vi "Global_Pictures.vi"() -> ()   [LabVIEW 2010]
panel:
  in  "sw PF Dir":bool[](array[boolean])
  in  "Tr PF Dir":bool[](array[boolean])
  in  "Line PF Dir":bool[](array[boolean])
  in  "Selection":bool
  in  "Zoom Delta":dbl
  in  "Layer History":string[](array[string])
  in  "Selected Layer":string
  out "ColorScale":picture
  in  "Tr Colors":u32[](array[colorbox])
  in  "sw Colors":u32[](array[colorbox])
  in  "Tr names":string[](array[string])
  in  "sw names":string[](array[string])
  in  "Init Idx":i32
  in  "Init Coords":cluster{"X":i32, "Y":i32}
  in  "Latest Element":string[](array[string])
  in  "Zoom Mini":dbl
  in  "Color":u32(colorbox)=6618880
  in  "Temp_Color":bool
  in  "Layer":string
  in  "Zoom":bool
  in  "Update GUI":bool
  in  "Line Colors":u32[](array[colorbox])
  in  "Line names":string[](array[string])
  in  "Color mode":T1(ring)
  in  "Zoom Factor":dbl
  in  "Last Position":cluster{"X":i32, "Y":i32}
  in  "Temp_4":refnum<vi>
  in  "Remove Grid":bool
  in  "Gb Reference":refnum<vi>
  out "Pictures":picture[](array[picture])
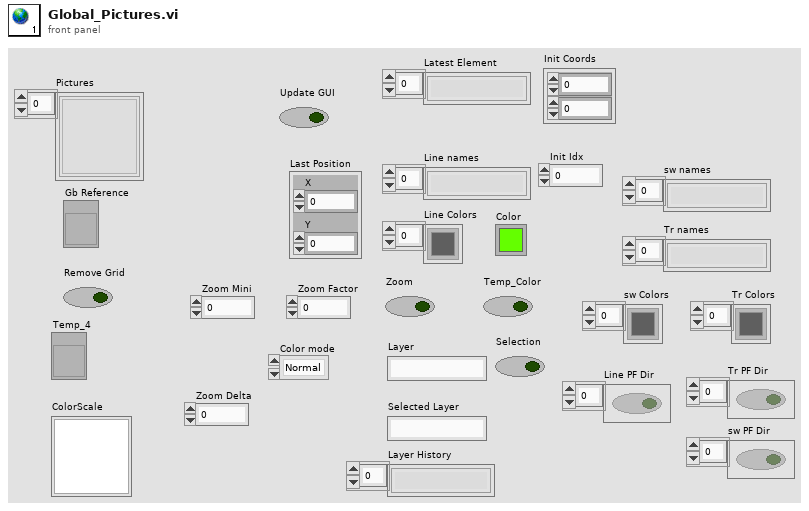
[diagram p1: front panel]
types:
  T1 = enum16{"Normal", "Power", "Isolated", "Emergency"}
diagram:
